vi "single sweep - next chunk - V0.vi"(4 "algorithm":string="statemachine", 5 "cursor bracket: Scan, win":refnum<vi>, 6 "mode":enum16{"first time", "uniform", "adaptive"}(ring)=enum."adaptive", 7 "Plot:response":refnum<vi>, 9 "x + iy":cdb[](array[numeric])=[0.0014961444378751654-0.005494848789731022i, 0.0014279223595474386-0.005470747752736027i, 0.001513711413730512-0.00552874878044623i, 0.001502407562898675-0.005445638194888334i, 0.0015845696982058808-0.005437153149732619i, 0.0015101628497750257-0.005522728337901211i, 0.0015131031857027845-0.005520920485579818i, 0.0015751707865244427-0.005432155579139866i, 0.001381283887581937-0.0055376532176146485i, 0.0013869914972504977-0.005471269712968517i], 10 "chunks":T1={"start F"=1400000.0, "stop F"=3000000.0, "total number of points"=6000, "chunk size"=10, "freq step (Hz)"=400.0, "update rate (Hz)"=250.0, "adaptive parameters"={"wavepacket"={"R"=0.5, "wave number"=15.0, "delta k"=7.0, "radii vector"=[], "radial section"=[], "wave vector"=22.0, "wavepacket is"=TRUE}, "number of grid points"=50, "decimation threshold"=1, "Voltage range"=0.1, "target freq step"=20.0, "target spot size"=0.05, "factor"=1.0, "another factor"=1.0, "analyze last # sec"=1, "scale factor"=10}, "total sweep time (sec)"=24.0, "chunk time (sec)"=0.04, "spot size (V)"=5.8152639158694506e-05, "uniform freq step (Hz)"=266.6666666666667, "next start freq"=1412960.0000000002} {"next start freq" format="%#_4f"; "uniform freq step (Hz)" format="%#_3f"; "spot size (V)" format="%#_2f"; "adaptive parameters"."wavepacket"."delta k" format="%#_3f"; "adaptive parameters"."wavepacket"."wave number" format="%#_3f"; "adaptive parameters"."wavepacket"."R" format="%#_3f"; "freq step (Hz)" format="%#_2f"; "stop F" format="%#_3f"; "start F" format="%#_3f"}, 11 "F Array in":dbl[](array[numeric])=[1408640.0000000002, 1408672.0000000002, 1408704.0000000002, 1408736.0000000002, 1408768.0000000002, 1408800.0000000002, 1408832.0000000002, 1408864.0000000002, 1408896.0000000002, 1408928.0000000002]) -> (0 "window":cluster{dbl[], dbl[]}[](array[cluster])=[{array[500 elements], array[500 elements]}, {array[500 elements], array[500 elements]}, {[2988000.0, 2988320.0, 2988640.0, 2992640.0, 2996640.0, 3000640.0, 3004640.0, 3004960.0, 3008960.0, 3012960.0, 3013280.0, 3013600.0, 3017600.0, 3021600.0, 3025600.0, 3029600.0, 3033600.0, 3037600.0, 3041600.0, 3045600.0, 3049600.0, 3053600.0, 3057600.0, 3061600.0, 3065600.0, 3069600.0, 3073600.0, 3077600.0, 3077920.0, 3081920.0, 3085920.0, 3089920.0, 3093920.0, 3094240.0, 3098240.0, 3102240.0, 3102560.0, 3106560.0, 3110560.0, 3114560.0, 3118560.0, 3122560.0, 3126560.0, 3126880.0, 3130880.0, 1408320.0000000002, 1408640.0000000002, 1408960.0000000002, 1412960.0000000002, 1416960.0000000002], [0.00011132389559019453, 0.00010071650784182846, 0.00011473215051580125, 0.00014782978553753255, 0.00012363182181742826, 8.247818640394286e-05, 4.853569183607435e-05, 0.00011091209952173231, 5.335161099533373e-05, 8.997863187674346e-05, 6.096859045620223e-05, 0.00011032129342938127, 0.00014137261844608594, 0.00011027777124700277, 7.83124094059187e-05, 8.359930932665522e-05, 8.923138939621333e-05, 5.1551353463386254e-05, 8.295869472945261e-05, 8.128556971740557e-05, 7.69462000730066e-05, 7.144851315975473e-05, 7.952519321081926e-05, 9.517779850815267e-05, 9.704248606160299e-05, 0.00011632633414436816, 0.00010390576558171027, 0.00010696411213824573, 9.728970607203878e-05, 0.0001308279684608251, 6.464132471543712e-05, 0.00011952708368690759, 6.148514772660781e-05, 8.068062707804084e-05, 0.00011312139911462234, 6.908047023895298e-05, 5.936822230667681e-05, 0.00010020626764101784, 0.00012946703718681504, 0.00010013466000813908, 6.912354981532708e-05, 0.00011430443059521424, 0.00012513022719631484, 0.00010923915541343698, 0.00011547570124367561, 0.003905008531492904, 0.0033917347983675613, 0.003353407371274829, 0.003173893478063239, 0.003074549188462509]}, {[2988000.0, 2988320.0, 2988640.0, 2992640.0, 2996640.0, 3000640.0, 3004640.0, 3004960.0, 3008960.0, 3012960.0, 3013280.0, 3013600.0, 3017600.0, 3021600.0, 3025600.0, 3029600.0, 3033600.0, 3037600.0, 3041600.0, 3045600.0, 3049600.0, 3053600.0, 3057600.0, 3061600.0, 3065600.0, 3069600.0, 3073600.0, 3077600.0, 3077920.0, 3081920.0, 3085920.0, 3089920.0, 3093920.0, 3094240.0, 3098240.0, 3102240.0, 3102560.0, 3106560.0, 3110560.0, 3114560.0, 3118560.0, 3122560.0, 3126560.0, 3126880.0, 3130880.0, 1408320.0000000002, 1408640.0000000002, 1408960.0000000002, 1412960.0000000002, 1416960.0000000002], [0.013694694005932529, 0.014489837272950239, 0.009503558469975002, 0.009528211653947193, 0.012476459558180022, 0.013578618032833986, 0.020768560303619083, 0.020949019291147796, 0.02034486055557658, 0.011646926818591538, 0.009458678658119484, 0.006310537358577627, 0.00038583342676350336, 0.006103250811137311, 0.001250242454873757, 0.005243640192020321, 0.008719705117003948, 0.006143859432854482, 0.006470257084291946, 0.006348276391260311, 0.008375758813583493, 0.0038044691071716097, 0.0015818509944146705, 0.003581191521982118, 0.0006892804064302445, 0.0025054554152808646, 0.004117073317010084, 0.002045540413627015, 0.0007410657254269008, 0.005324792655608368, 0.012491486267365477, 0.013829845176253889, 0.009382411909246033, 0.008531253899751555, 0.006057094794442862, 0.000802518050976467, 0.006846069080773061, 0.004537353265510852, 0.008159903085244793, 0.0028444703551188284, 0.007454427723095375, 4.4410190171195404e-05, 0.0015101954709487865, 0.004475681662266171, 0.010341490132182555, 0.01226244459723875, 0.015308020505903021, 0.005597683037877003, 0.0037965342629815418, 0.0016913227005998597]}], 1 "fancy circles":cluster{dbl[], dbl[]}[](array[cluster])=[{[0.004347976639836461, 0.0043237329011621035, 0.004251384023380436, 0.004132070991513198, 0.003967675443347089, 0.0037607899948818246, 0.0035146773532270816, 0.00323321886176232, 0.0029208532890330928, 0.002582506826719488, 0.00222351540065057, 0.0018495405200665291, 0.0014664799922359413, 0.001080374910511962, 0.0006973143826813736, 0.0003233395020973332, -3.56519239715844e-05, -0.0003739983862851902, -0.0006863639590144167, -0.0009678224504791784, -0.0012139350921339205, -0.0014208205405991845, -0.001585216088765295, -0.0017045291206325324, -0.0017768779984142003, -0.001801121737088557, -0.0017768779984142003, -0.0017045291206325324, -0.0015852160887652941, -0.001420820540599184, -0.00121393509213392, -0.000967822450479178, -0.0006863639590144162, -0.00037399838628518847, -3.5651923971582664e-05, 0.0003233395020973332, 0.0006973143826813741, 0.0010803749105119625, 0.0014664799922359426, 0.001849540520066531, 0.0022235154006505697, 0.002582506826719488, 0.0029208532890330936, 0.003233218861762321, 0.003514677353227083, 0.0037607899948818254, 0.003967675443347089, 0.004132070991513199, 0.004251384023380437, 0.0043237329011621035], [-0.00253283204245687, -0.0021474888509143563, -0.001768222751695333, -0.0014010149977470693, -0.0010516566747086093, -0.0007256573720308159, -0.00042815829345946126, -0.00016385117718095135, 6.309569569158376e-05, 0.0002491032374014545, 0.0003912379979003752, 0.0004872584271080889, 0.0005356502254961651, 0.0005356502254961651, 0.00048725842710808844, 0.0003912379979003752, 0.00024910323740145405, 6.309569569158376e-05, -0.00016385117718095135, -0.0004281582934594617, -0.0007256573720308154, -0.0010516566747086097, -0.00140101499774707, -0.0017682227516953328, -0.0021474888509143567, -0.002532832042456871, -0.002918175233999384, -0.003297441333218408, -0.003664649087166672, -0.004014007410205131, -0.004340006712882925, -0.004637505791454279, -0.004901812907732789, -0.005128759780605325, -0.005314767322315195, -0.005456902082814115, -0.0055529225120218295, -0.005601314310409906, -0.005601314310409906, -0.005552922512021829, -0.005456902082814115, -0.005314767322315195, -0.0051287597806053235, -0.004901812907732788, -0.004637505791454277, -0.004340006712882922, -0.004014007410205131, -0.0036646490871666704, -0.0032974413332184063, -0.0029181752339993822]}, {[-0.0007985969840225416, -0.0005913945404828922, -0.0003841920969432428, -0.0001769896534035934, 3.0212790136055923e-05, 0.00023741523367570524, 0.0004446176772153548, 0.0006518201207550041, 0.0008590225642946534, 0.0010662250078343027, 0.001273427451373952, 0.0014806298949136016, 0.001687832338453251, 0.0018950347819929002, 0.00210223722553255, 0.0023094396690721986, 0.002516642112611848, 0.0027238445561514977, 0.0029310469996911472, 0.003138249443230796], [-0.004804300169328853, -0.004577153356641655, -0.004350006543954456, -0.004122859731267258, -0.00389571291858006, -0.0036685661058928616, -0.003441419293205663, -0.003214272480518465, -0.0029871256678312666, -0.002759978855144068, -0.00253283204245687, -0.0023056852297696716, -0.002078538417082473, -0.0018513916043952751, -0.0016242447917080766, -0.0013970979790208786, -0.0011699511663336801, -0.0009428043536464817, -0.0007156575409592832, -0.0004885107282720852]}, {[-0.0009980406754980312, -0.0007708938628108329, -0.0005437470501236345, -0.0003166002374364362, -8.945342474923792e-05, 0.00013769338793796033, 0.0003648402006251588, 0.0005919870133123571, 0.0008191338259995553, 0.0010462806386867538, 0.0012734274513739518, 0.0015005742640611503, 0.0017277210767483488, 0.001954867889435547, 0.0021820147021227453, 0.0024091615148099433, 0.002636308327497142, 0.0028634551401843403, 0.0030906019528715387, 0.0033177487655587368], [-0.0004608076070603765, -0.0006680100506000258, -0.0008752124941396752, -0.0010824149376793247, -0.001289617381218974, -0.0014968198247586233, -0.0017040222682982728, -0.0019112247118379222, -0.0021184271553775715, -0.0023256295989172206, -0.00253283204245687, -0.0027400344859965196, -0.002947236929536169, -0.0031544393730758183, -0.003361641816615468, -0.003568844260155117, -0.0037760467036947664, -0.003983249147234416, -0.004190451590774065, -0.004397654034313714]}], 2 "chunks out":T1={"start F"=1400000.0, "stop F"=3000000.0, "total number of points"=6000, "chunk size"=10, "freq step (Hz)"=400.0, "update rate (Hz)"=250.0, "adaptive parameters"={"wavepacket"={"R"=0.5, "wave number"=15.0, "delta k"=7.0, "radii vector"=[], "radial section"=[], "wave vector"=22.0, "wavepacket is"=TRUE}, "number of grid points"=50, "decimation threshold"=1, "Voltage range"=0.1, "target freq step"=20.0, "target spot size"=0.05, "factor"=1.0, "another factor"=1.0, "analyze last # sec"=1, "scale factor"=10}, "total sweep time (sec)"=24.0, "chunk time (sec)"=0.04, "spot size (V)"=5.8152639158694506e-05, "uniform freq step (Hz)"=266.6666666666667, "next start freq"=1412960.0000000002} {"next start freq" format="%#_4f"; "uniform freq step (Hz)" format="%#_3f"; "spot size (V)" format="%#_2f"; "adaptive parameters"."wavepacket"."delta k" format="%#_3f"; "adaptive parameters"."wavepacket"."wave number" format="%#_3f"; "adaptive parameters"."wavepacket"."R" format="%#_3f"; "freq step (Hz)" format="%#_2f"; "stop F" format="%#_3f"; "start F" format="%#_3f"}, 3 "F Array":dbl[](array[numeric])=[1412960.0000000002, 1413360.0000000002, 1413760.0000000002, 1414160.0000000002, 1414560.0000000002, 1414960.0000000002, 1415360.0000000002, 1415760.0000000002, 1416160.0000000002, 1416560.0000000002])   [LabVIEW 2010]
uses:
  single sweep - frequency chunks.ctl
  single sweep - adaptive parameters.ctl
  wavepacket.ctl
  generate wave packet V2.vi
  smart decimate .vi
  set up complex region.vi
  inteference -- find center V2.vi
  find circle corners V3.vi
  linear interpolation - re.vi
  peak - phase around center.vi
  peak - simple guess at omega.vi
  peak - fix phase.vi
  peak - fit phase around center.vi
  peak - calculate lorentzian.vi
  draw a line.vi
  draw a circle.vi
  generate linear region.vi
  find circle corners - rescale back.vi
  <vilib>/Analysis/baseanly.llb/Median.vi
  <vilib>/Analysis/baseanly.llb/Mean.vi
  <vilib>/Analysis/2dsp.llb/Unwrap Phase.vi
  <vilib>/gmath/NumericalOptimization/Nonlinear Curve Fit.vi
  <vilib>/gmath/NumericalOptimization/Nonlinear Curve Fit LM.vi
  <vilib>/Utility/error.llb/Clear Errors.vi
panel:
  in  "in peak win (kHz)":dbl=0.5
  in  "in peak threshold":i32=10
  in  "search win (kHz)":dbl=12.0
  in  "scale factor":i32=3
  out "in peak threshold  ?":bool
  in  "analyze last # of secs":dbl=0.3
  out "omega(0) (kHz)":dbl=3120.5599996327037 format="%#_4f"
  in  "min speed (kHz/sec)":dbl=8.0
  in  "max speed (kHz/sec)":dbl=100.0
  out "thershold ?":bool=TRUE
  in  "threshold":dbl=20.0
  out "heater":dbl=5.77997331934377
  out "ln(x) 0":dbl=-6.907755278982137
  out "ln(x)":dbl=-9.498835202893684
  in  "negative":i32=2
  in  "I (sec)":dbl=2.0
  in  "dz0":dbl=0.001 format="%#_6f"
  in  "max dF":dbl=2000.0
  in  "min dF":dbl=20.0
  in  "P":dbl=2.0
  out "32bit integer":i32=50
  out "above ?":bool
  in  "V":dbl=0.05
  in  "factor":dbl=0.8
  out "r":dbl
  out "viscosity":dbl
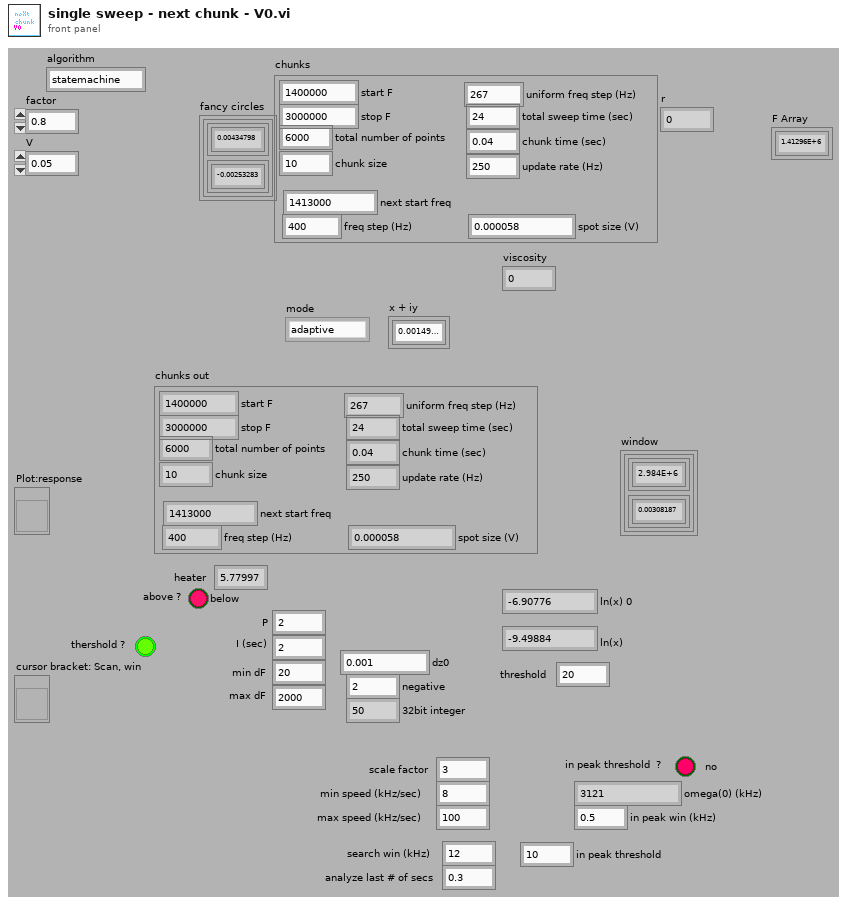
[diagram p1: front panel]
types:
  T1 = typedef "single sweep - frequency chunks.ctl" = cluster{"start F":dbl, "stop F":dbl, "total number of points":i32, "chunk size":i32, "freq step (Hz)":dbl, "update rate (Hz)":dbl, "adaptive parameters":T2, "total sweep time (sec)":dbl, "chunk time (sec)":dbl, "spot size (V)":dbl, "uniform freq step (Hz)":dbl, "next start freq":dbl}
  T2 = typedef "single sweep - adaptive parameters.ctl" = cluster{"wavepacket":T3, "number of grid points":i32, "decimation threshold":i32, "Voltage range":dbl, "target freq step":dbl, "target spot size":dbl, "factor":dbl, "another factor":dbl, "analyze last # sec":i32, "scale factor":i32}
  T3 = typedef "wavepacket.ctl" = cluster{"R":dbl, "wave number":dbl, "delta k":dbl, "radii vector":dbl[], "radial section":cdb[], "wave vector":dbl, "wavepacket is":bool}
  T4 = enum16{"", "cursor moves", "center change", "window change", "init", "check", "reset", "set y to middle"}
  T5 = typedef "circle corners.ctl" = cluster{"z (-pi/2)":cdb, "z(inf)":cdb, "z (pi/2)":cdb, "z center":cdb, "z(0)":cdb, "radius":dbl}
  T6 = typedef "lorentzian.ctl" = cluster{"Amplitude":dbl, "omega(0)":dbl, "Gamma":dbl, "phase":dbl, "Q":dbl, "Norm  Ampl":dbl, "z (inf)":cdb, "4corners":T5}
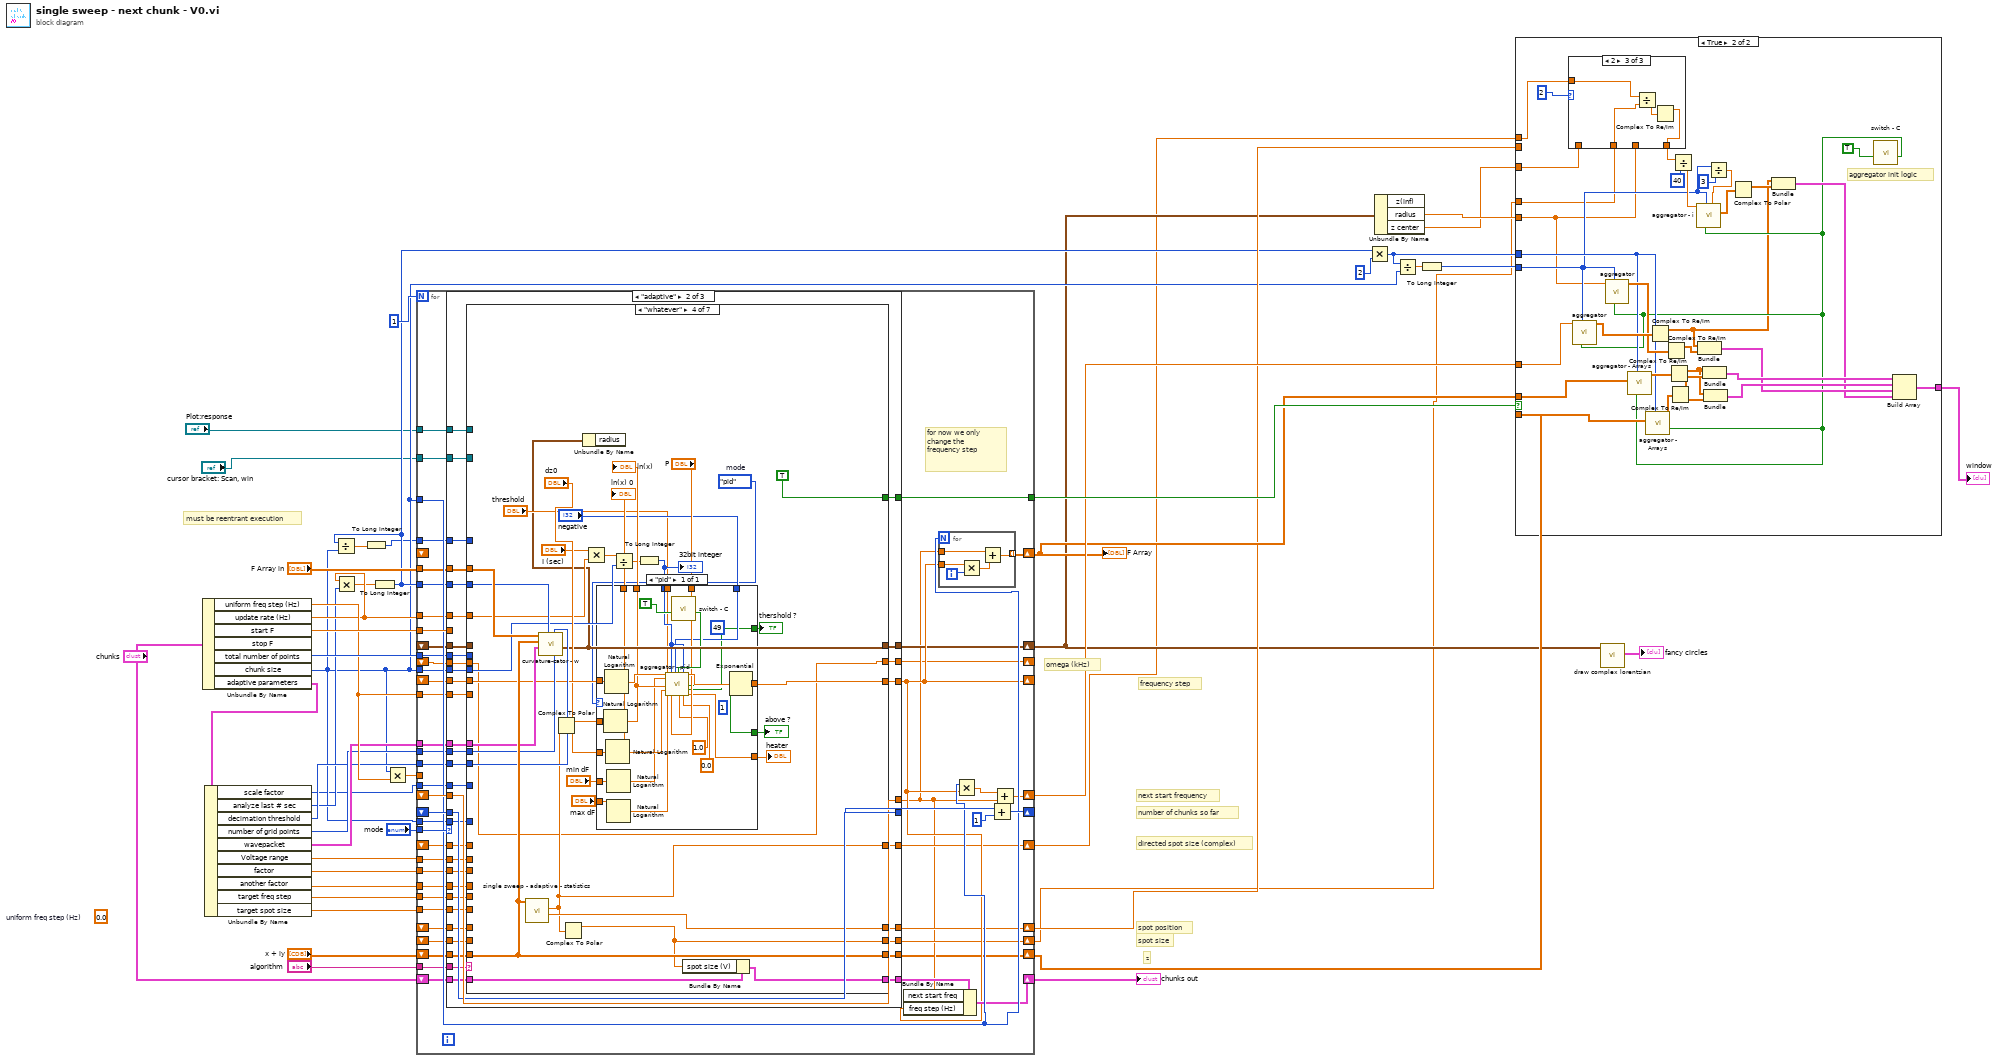
[diagram p0: block diagram]
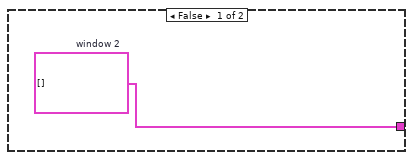
[diagram p2: hidden frame]
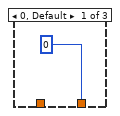
[diagram p3: hidden frame]
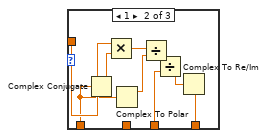
[diagram p4: hidden frame]
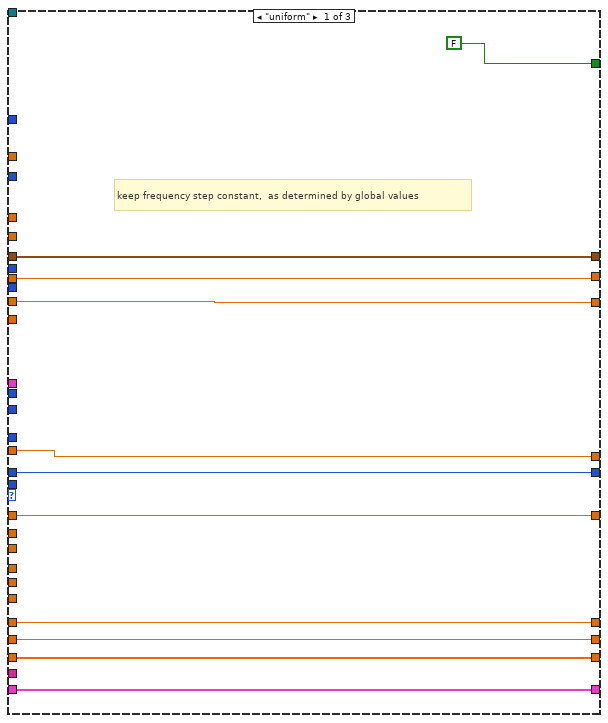
[diagram p5: hidden frame]
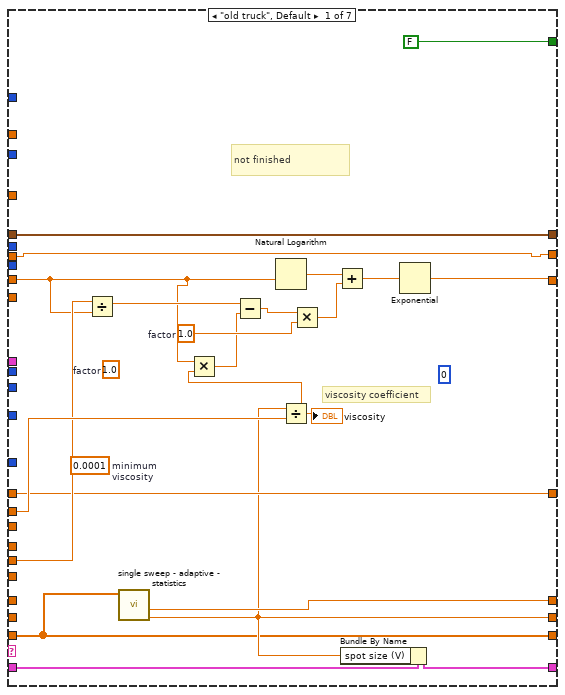
[diagram p6: hidden frame]
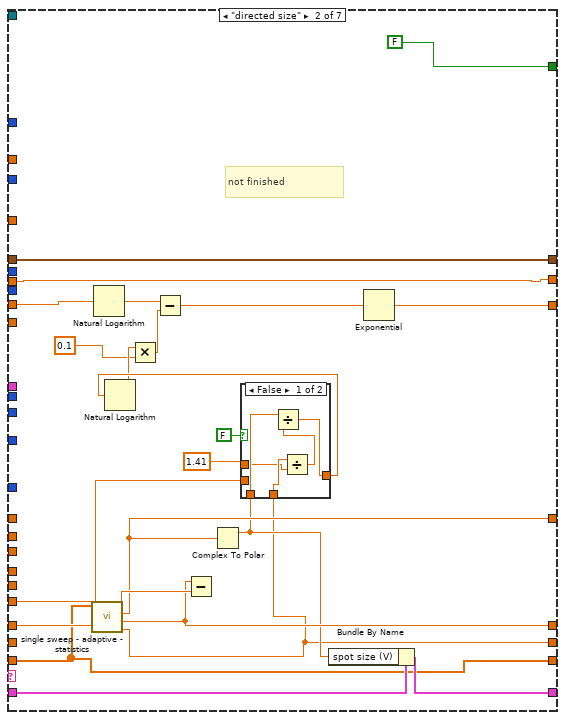
[diagram p7: hidden frame]
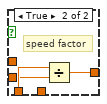
[diagram p8: hidden frame]
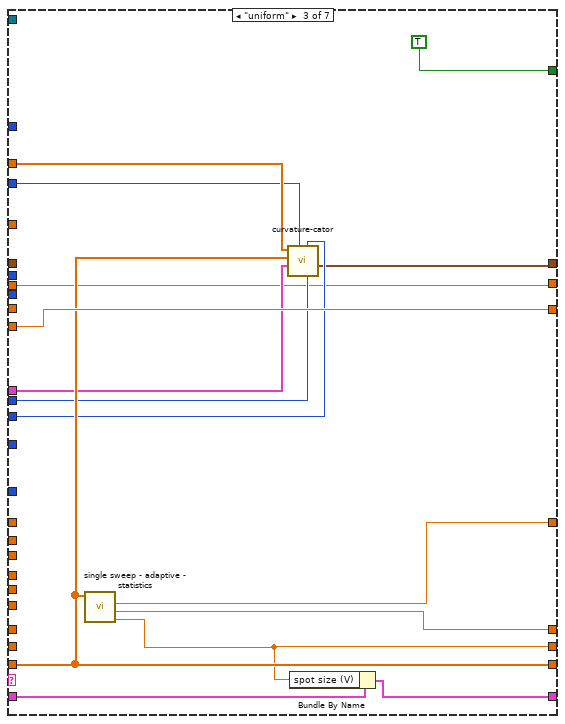
[diagram p9: hidden frame]
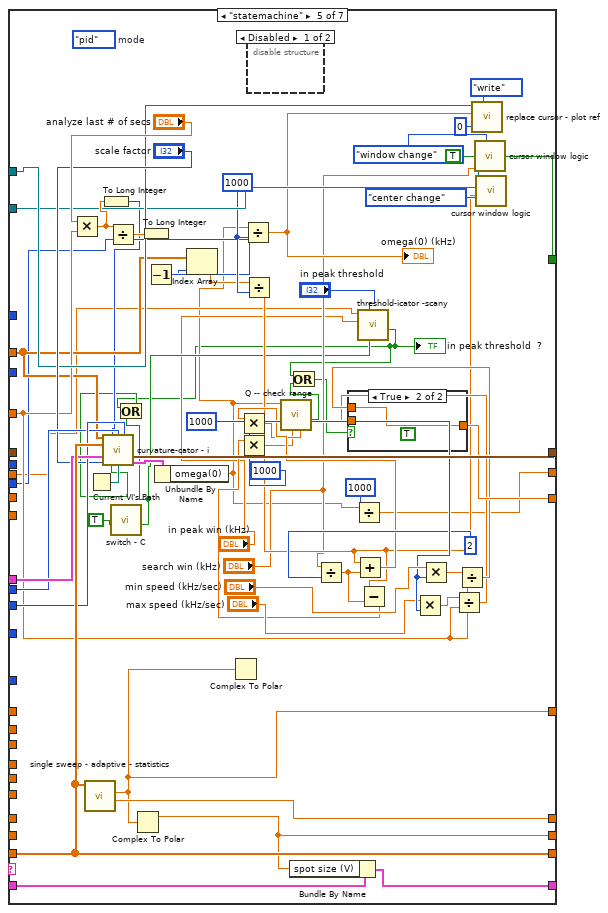
[diagram p10: hidden frame]
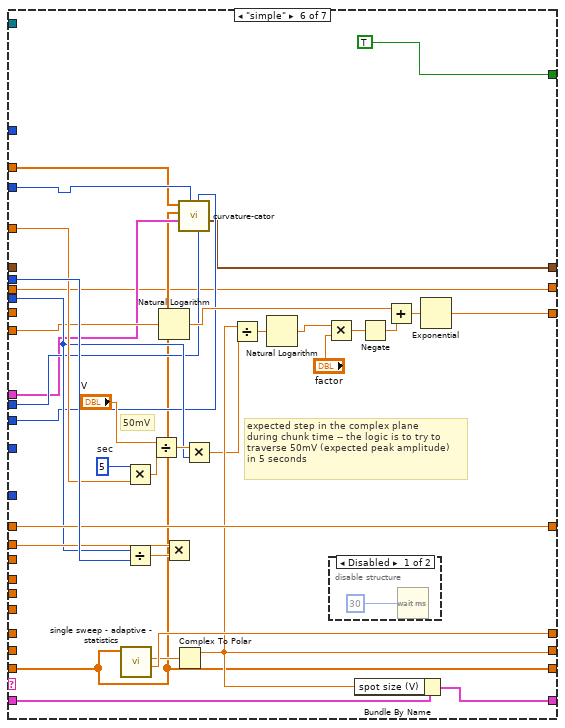
[diagram p13: hidden frame]
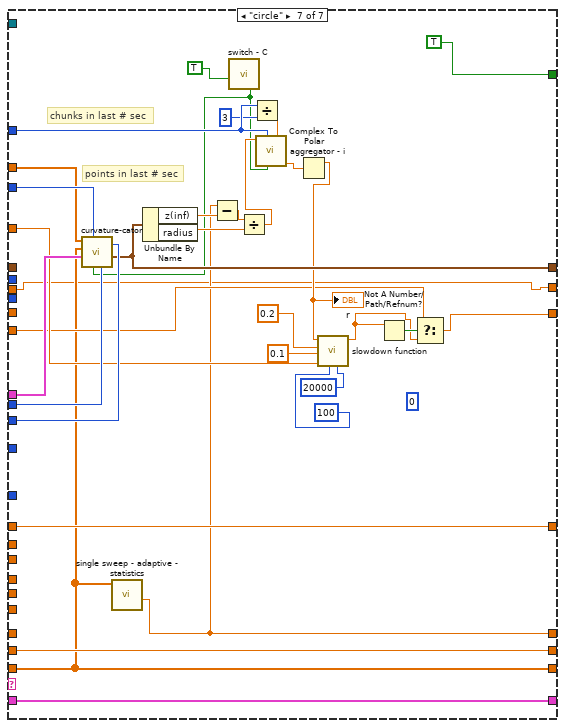
[diagram p15: hidden frame]
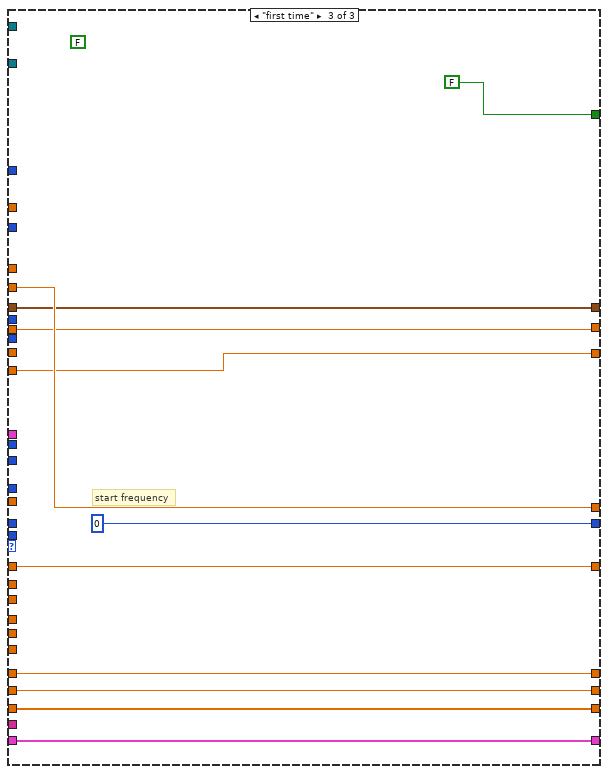
[diagram p16: hidden frame]
diagram:
  (unwired) 0.0  # uniform freq step (Hz)
  # "omega (kHz)"
  # "z"
  # "must be reentrant execution"
  # "directed spot size (complex)"
  # "spot position"
  # "spot size"
  # "frequency step"
  # "number of chunks so far"
  # "next start frequency"
  n1 = Unbundle By Name("chunks") -> ("uniform freq step (Hz)"=w31:dbl, "update rate (Hz)"=w29:dbl, "start F"=w44:dbl, "total number of points"=w40:i32, "chunk size"=w11:i32, "adaptive parameters"=w37:T2)  [unwired: 1 out]
  n2 = Unbundle By Name(w37) -> ("scale factor"=w3:i32, "analyze last # sec"=w25:i32, "decimation threshold"=w26:i32, "number of grid points"=w27:i32, "wavepacket"=w28:T3, "Voltage range"=w33:dbl, "factor"=w35:dbl, "another factor"=w34:dbl, "target freq step"=w36:dbl, "target spot size"=w32:dbl)
  n3 = Multiply(x=w29, y=w25) -> (x*y=w23:dbl)
  n4 = To Long Integer(number=w23) -> (32bit integer=w12:i32)
  n5 = Divide(x=w12, y=w11) -> (x/y=w10:dbl)
  n6 = To Long Integer(number=w10) -> (32bit integer=w9:i32)
  n7 = Multiply(x=w11, y=w31) -> (x*y=w45:dbl)
  n8 = for {
    N: 1 -> [_]
    tunnel: w31 -> [w66]
    tunnel: w11 -> [w88]
    tunnel: "mode" -> [w96]
    shift-right: [w56] -> w22
    shift-left: _ -> [w94]
    shift-right: [w91] -> _
    shift-left: _ -> [w93]
    tunnel: w45 -> [_]
    tunnel: w44 -> [w89]
    shift-right: [w95] -> w20
    shift-left: _ -> [_]
    tunnel: "F Array in" -> [w85]
    tunnel: w11 -> [w84]
    tunnel: w40 -> [w83]
    tunnel: w33 -> [w82]
    shift-right: [w81] -> w39
    shift-left: "chunks" -> [w76]
    shift-right: [w80] -> _
    shift-left: _ -> [w79]
    tunnel: "algorithm" -> [w78]
    tunnel: w36 -> [w77]
    shift-right: [w74] -> w4
    shift-left: _ -> [w71]
    shift-right: [w73] -> w13
    shift-left: _ -> [w72]
    tunnel: w11 -> [w70]
    shift-right: [w69] -> w6
    shift-left: _ -> [w67]
    tunnel: w32 -> [w68]
    tunnel: w35 -> [w65]
    tunnel: w34 -> [w64]
    tunnel: w29 -> [w63]
    tunnel: w12 -> [w62]
    tunnel: w28 -> [w61]
    tunnel: w27 -> [w60]
    tunnel: w26 -> [w59]
    shift-right: [w58] -> w7
    shift-left: _ -> [w57]
    tunnel: [w53] -> w24
    shift-right: [w54] -> w18
    shift-left: "x + iy" -> [w86]
    tunnel: w9 -> [w52]
    tunnel: w3 -> [w51]
    tunnel: "cursor bracket: Scan, win" -> [w50]
    tunnel: "Plot:response" -> [w49]
    shift-right: [w48] -> _
    shift-left: _ -> [w47]
    # "for now we only change the \nfrequency step"
    n9 = case shown="\"adaptive\"" w96 {
      tunnel: [w107 w146 w411] -> w55
      tunnel: [w105 w145 0] -> w92
      tunnel: w94 -> [w107 w146 _]
      tunnel: w93 -> [w105 w145 _]
      tunnel: w89 -> [_ _ w411]
      tunnel: [w106 w143 w406] -> w80
      tunnel: w79 -> [w106 w144 _]
      tunnel: w86 -> [w98 w142 w403]
      tunnel: w85 -> [_ w141 _]
      tunnel: w84 -> [_ w140 _]
      tunnel: w83 -> [_ w139 _]
      tunnel: w82 -> [_ w138 _]
      tunnel: w78 -> [_ w137 _]
      tunnel: w77 -> [_ w136 _]
      tunnel: w76 -> [w104 w135 w410]
      tunnel: [w104 w134 w410] -> w75
      tunnel: [w102 w133 w408] -> w74
      tunnel: [w103 w132 w409] -> w73
      tunnel: w72 -> [w103 w131 w409]
      tunnel: w71 -> [w102 w130 w408]
      tunnel: w70 -> [_ w129 _]
      tunnel: [w101 w128 w407] -> w69
      tunnel: w68 -> [_ w127 _]
      tunnel: w67 -> [w101 w126 w407]
      tunnel: w66 -> [_ w123 w406]
      tunnel: w65 -> [_ w125 _]
      tunnel: w64 -> [_ w124 _]
      tunnel: w63 -> [_ w122 _]
      tunnel: w62 -> [_ w121 _]
      tunnel: w61 -> [_ w120 _]
      tunnel: w60 -> [_ w119 _]
      tunnel: w59 -> [_ w118 _]
      tunnel: [w100 w117 w405] -> w58
      tunnel: w57 -> [w100 w116 w405]
      tunnel: [FALSE w115 FALSE] -> w53
      tunnel: [w98 w114 w403] -> w54
      tunnel: w52 -> [_ w113 _]
      tunnel: w51 -> [_ w112 _]
      tunnel: w50 -> [_ w111 _]
      tunnel: w49 -> [_ w110 _]
      tunnel: [w97 w109 w402] -> w48
      tunnel: w47 -> [w97 w108 w402]
      frame "uniform" {
        # "keep frequency step constant,  as determined by global values"
      }
      frame "adaptive" {
        n10 = case shown="\"whatever\"" w137 {
          tunnel: w144 -> [w154 w180 _ w238 _ _ _]
          tunnel: [w157 w179 w212 w237 w317 w351 w373] -> w143
          tunnel: w142 -> [w148 w169 w208 w245 w330 w336 w372]
          tunnel: w141 -> [_ _ w209 w246 w288 w340 w397]
          tunnel: w140 -> [_ _ _ w225 w286 w353 _]
          tunnel: w139 -> [_ _ _ _ _ w366 _]
          tunnel: w138 -> [w163 _ _ _ _ w365 _]
          tunnel: w136 -> [w162 _ _ _ _ _ _]
          tunnel: w135 -> [w165 w189 w199 w239 w324 w363 w401]
          tunnel: [w164 w188 w200 w240 w325 w364 w401] -> w134
          tunnel: [w151 w174 w201 w231 w322 w359 w400] -> w133
          tunnel: [w152 w186 w211 w247 w331 w361 w371] -> w132
          tunnel: w131 -> [_ w187 _ _ _ _ _]
          tunnel: w130 -> [_ _ _ _ _ _ w400]
          tunnel: w129 -> [_ _ _ _ _ _ _]
          tunnel: [w153 w185 w210 w232 w323 w362 w399] -> w128
          tunnel: w127 -> [_ w183 _ _ _ _ _]
          tunnel: w126 -> [w153 _ _ _ _ w362 w399]
          tunnel: w125 -> [_ _ _ _ _ _ _]
          tunnel: w124 -> [_ _ _ _ _ _ _]
          tunnel: w123 -> [_ _ w212 _ _ w344 w374]
          tunnel: w122 -> [_ _ _ w222 w298 w357 w382]
          tunnel: w121 -> [_ _ w204 w226 _ w341 w398]
          tunnel: w120 -> [_ _ w207 w244 w329 w339 w396]
          tunnel: w119 -> [_ _ w205 w242 w327 w342 w395]
          tunnel: w118 -> [_ _ w206 w243 w328 w343 w394]
          tunnel: [w150 w171 w202 w216 w320 w338 w388] -> w117
          tunnel: w116 -> [w150 w171 _ _ _ _ _]
          tunnel: [FALSE FALSE TRUE TRUE TRUE TRUE TRUE] -> w115
          tunnel: [w148 w169 w208 w245 w330 w336 w372] -> w114
          tunnel: w113 -> [_ _ _ _ _ _ w391]
          tunnel: w112 -> [_ _ _ _ _ _ _]
          tunnel: w111 -> [_ _ _ _ w310 _ _]
          tunnel: w110 -> [_ _ _ _ w313 _ _]
          tunnel: [w147 w168 w198 w213 w274 w334 w369] -> w109
          tunnel: w108 -> [w147 w168 w198 w213 w279 w334 w369]
          frame "old truck", Default {
            (unwired) 0
            (unwired) 1.0  # factor
            w160 = 1.0  # factor
            (unwired) 0.0001  # minimum  viscosity
            # "not finished"
            # "viscosity coefficient"
            n11 = Divide(x=w162, y=w154) -> (x/y=w161:dbl)
            n12 = call "single sweep - adaptive - statistics.vi"("x + iy"=w148) -> ("spot size"=w151:dbl, "spot position"=w152:cdb)  [unwired: 8 in, 1 out]
            n13 = Natural Logarithm(1:w154) -> (0:w159:dbl)
            n14 = Divide(x=w151, y=w163) -> (x/y=w156:dbl)
            "viscosity" <- w156
            n15 = Multiply(x=w154, y=w156) -> (x*y=w155:dbl)
            n16 = Subtract(x=w161, y=w155) -> (x-y=w167:dbl)
            n17 = Multiply(x=w167, y=w160) -> (x*y=w166:dbl)
            n18 = Add(x=w159, y=w166) -> (x+y=w158:dbl)
            n19 = Bundle By Name(cluster=w165, "spot size (V)"=w151) -> (w164:T1)
            n20 = Exponential(1:w158) -> (0:w157:dbl)
          }
          frame "directed size" {
            # "not finished"
            n21 = call "single sweep - adaptive - statistics.vi"("x + iy"=w169) -> ("spot size"=w174:dbl, "spot position"=w186:cdb, "spot directed size"=w185:cdb)  [unwired: 8 in]
            n22 = Natural Logarithm(1:w180) -> (0:w182:dbl)
            n23 = Subtract(x=w186, y=w187) -> ()  [unwired: 1 out]
            n24 = Complex To Polar(r * e^(i*theta)=w185) -> (r=w184:dbl)  [unwired: 1 out]
            n25 = case shown="False" FALSE {
              tunnel: w184 -> [w194 w197]
              tunnel: w183 -> [_ w196]
              tunnel: [w193 w195] -> w178
              tunnel: w174 -> [w192 _]
              tunnel: 1.41 -> [w190 _]
              frame False {
                n26 = Divide(x=w192, y=w190) -> (x/y=w191:dbl)
                n27 = Divide(x=w194, y=w191) -> (x/y=w193:dbl)
              }
              frame True {
                # "speed factor"
                n28 = Divide(x=w197, y=w196) -> (x/y=w195:dbl)
              }
            }
            n29 = Natural Logarithm(1:w178) -> (0:w177:dbl)
            n30 = Multiply(x=w177, y=0.1) -> (x*y=w176:dbl)
            n31 = Subtract(x=w182, y=w176) -> (x-y=w181:dbl)
            n32 = Bundle By Name(cluster=w189, "spot size (V)"=w184) -> (w188:T1)
            n33 = Exponential(1:w181) -> (0:w179:dbl)
          }
          frame "uniform" {
            n34 = call "single sweep - adaptive - statistics.vi"("x + iy"=w208) -> ("spot size"=w201:dbl, "spot position"=w211:cdb, "spot directed size"=w210:cdb)  [unwired: 8 in]
            n35 = call "curvature-cator.vi"("number of grid points"=w205, "decimation threshold"=w206, "size"=w204, "wavepacket in"=w207, "z array in"=w208, "omega array in"=w209) -> ("4 corners out"=w202:T5)  [unwired: 3 in, 2 out]
            n36 = Bundle By Name(cluster=w199, "spot size (V)"=w201) -> (w200:T1)
          }
          frame "whatever" {
            w214 = enum16{"pid"}."pid"  # mode
            n37 = call "single sweep - adaptive - statistics.vi"("x + iy"=w245) -> ("spot position"=w247:cdb, "spot directed size"=w232:cdb)  [unwired: 8 in, 1 out]
            n38 = call "curvature-cator - w.vi"("number of grid points"=w242, "decimation threshold"=w243, "size"=w226, "wavepacket in"=w244, "z array in"=w245, "omega array in"=w246) -> ("4 corners out"=w216:T5)  [unwired: 3 in, 2 out]
            n39 = Complex To Polar(r * e^(i*theta)=w232) -> (r=w215:dbl)  [unwired: 1 out]
            n40 = Complex To Polar(r * e^(i*theta)=w232) -> (r=w231:dbl)  [unwired: 1 out]
            n41 = Unbundle By Name(w216) -> ()  [unwired: 1 out]
            n42 = Multiply(x="I (sec)", y=w222) -> (x*y=w221:dbl)
            n43 = Divide(x=w221, y=w225) -> (x/y=w227:dbl)
            n44 = To Long Integer(number=w227) -> (32bit integer=w224:i32)
            "32bit integer" <- w224
            n45 = case shown="\"pid\"" w214 {
              tunnel: w238 -> [w270]
              tunnel: [w267] -> w237
              tunnel: [w264] -> w236
              tunnel: "dz0" -> [w263]
              tunnel: [w262] -> w234
              tunnel: "P" -> [w261]
              tunnel: "min dF" -> [w259]
              tunnel: "max dF" -> [w258]
              tunnel: [w255] -> w228
              tunnel: w224 -> [w254]
              tunnel: "negative" -> [w252]
              tunnel: [w251] -> w219
              tunnel: "threshold" -> [w250]
              tunnel: [w249] -> w217
              tunnel: w215 -> [w248]
              frame "pid" {
                (unwired) 1 ("y")
                (unwired) 49 ("y")
                n46 = Natural Logarithm(1:w248) -> (0:w264:dbl)
                n47 = Natural Logarithm(1:w270) -> (0:w269:dbl)
                n48 = Natural Logarithm(1:w263) -> (0:w262:dbl)
                n49 = Natural Logarithm(1:w259) -> (0:w257:dbl)
                n50 = Natural Logarithm(1:w258) -> (0:w256:dbl)
                n51 = call "switch - C.vi"("switch"=TRUE) -> ("result"=w265:bool)  [unwired: 10 in]
                n52 = call "aggregator - pid.vi"("df"=w269, "low"=w257, "threshold"=w250, "dz"=w264, "dz0"=w262, "high"=w256, "requested size"=w254, "P"=w261, "negative"=w252, "first time"=w265, "I"=1.0 ("y"), "requested averaging interval"=w254, "D"=0.0 ("y")) -> ("new df"=w268:dbl, "above ?"=w255:bool, "thershold ?"=w249:bool, "heater"=w251:dbl)  [unwired: 3 in]
                n53 = Exponential(1:w268) -> (0:w267:dbl)
              }
            }
            "above ?" <- w228
            "ln(x)" <- w236
            "ln(x) 0" <- w234
            "heater" <- w219
            "thershold ?" <- w217
            n54 = Bundle By Name(cluster=w239, "spot size (V)"=w231) -> (w240:T1)
          }
          frame "statemachine" {
            w293 = 1000
            w300 = 1000
            w306 = 1000
            (unwired) enum16{"pid"}."pid"  # mode
            n55 = Multiply(x="analyze last # of secs", y=w298) -> (x*y=w315:dbl)
            n56 = call "single sweep - adaptive - statistics.vi"("x + iy"=w330) -> ("spot position"=w331:cdb, "spot directed size"=w323:cdb)  [unwired: 8 in, 1 out]
            n57 = Current VI's Path() -> (path=w319:path)
            n58 = To Long Integer(number=w315) -> (32bit integer=w284:i32)
            n59 = Divide(x=w315, y=w286) -> (x/y=w321:dbl)
            n60 = call "switch - C.vi"("switch"=TRUE) -> ("result"=w280:bool)  [unwired: 10 in]
            n61 = Complex To Polar(r * e^(i*theta)=w323) -> (r=w322:dbl)  [unwired: 1 out]
            n62 = To Long Integer(number=w321) -> ()  [unwired: 1 out]
            n63 = Decrement(x=w286) -> (x-1=w285:i32)
            n64 = Index Array(array=w288, index=w285) -> (element=w287:dbl)
            n65 = Complex To Polar(r * e^(i*theta)=w323) -> ()  [unwired: 2 out]
            n66 = Divide(x=w287, y=w306) -> (x/y=w289:dbl)
            n67 = disable-structure shown="Disabled" {
              frame Disabled {
              }
              frame Enabled {
              }
            }
            n68 = Bundle By Name(cluster=w324, "spot size (V)"=w322) -> (w325:T1)
            n69 = Divide(x="search win (kHz)", y=2) -> (x/y=w295:dbl)
            n70 = Add(x=w289, y=w295) -> (x+y=w294:dbl)
            n71 = Multiply(x=w294, y=w293) -> (x*y=w291:dbl)
            n72 = call "threshold-icator -scany.vi"("first time"=w280, "requested size"="in peak threshold", "gamma"="in peak win (kHz)", "omega"=w279) -> ("new peak"=w272:bool)  [unwired: 4 in, 3 out]
            "in peak threshold  ?" <- w272
            n73 = Or(x=w272, y=w280) -> (x .or. y?=w278:bool)
            n74 = call "curvature-cator - i.vi"("omega array in"=w288, "size"=w284, "number of grid points"=w327, "decimation threshold"=w328, "z array in"=w330, "wavepacket in"=w329, "scale factor"="scale factor", "first time"=w278, "main VI path"=w319) -> ("4 corners rescaled out"=w320:T5, "lorentzian out"=w318:T6)  [unwired: 3 in, 2 out]
            n75 = Unbundle By Name(w318) -> ("omega(0)"=w275:dbl)
            n76 = Divide(x=w275, y=w306) -> (x/y=w305:dbl)
            "omega(0) (kHz)" <- w305
            n77 = Divide(x=w275, y=1000) -> (x/y=w274:dbl)
            n78 = Subtract(x=w289, y=w295) -> (x-y=w292:dbl)
            n79 = Multiply(x=w292, y=w293) -> (x*y=w290:dbl)
            n80 = call "Q -- check range.vi"("upper"=w291, "lower"=w290, "number"=w275) -> ("in range?"=w273:bool)  [unwired: 4 in, 4 out]
            n81 = Or(x=w272, y=w273) -> (x .or. y?=w271:bool)
            n82 = Multiply(x="max speed (kHz/sec)", y=w300) -> (x*y=w301:dbl)
            n83 = Multiply(x="min speed (kHz/sec)", y=w300) -> (x*y=w303:dbl)
            n84 = Divide(x=w301, y=w298) -> (x/y=w297:dbl)
            n85 = Divide(x=w303, y=w298) -> (x/y=w302:dbl)
            n86 = case shown="True" w271 {
              tunnel: [w332 w333] -> w317
              tunnel: w302 -> [_ w333]
              tunnel: w297 -> [w332 _]
              frame False {
              }
              frame True {
                (unwired) TRUE
              }
            }
            n87 = call "replace cursor - plot ref.vi"("action"=enum16{"", "read", "write"}."write", "cursor index"=0, "new X"=w305, "Plot ref in"=w313) -> ()  [unwired: 5 in, 3 out]
            n88 = call "cursor window logic.vi"("action"=T4."center change", "center"=w289, "cursor bracket in"=w310) -> ("cursor bracket out"=w308:refnum<vi>)  [unwired: 7 in, 1 out]
            n89 = call "cursor window logic.vi"("action"=T4."window change", "window"="search win (kHz)", "cursor bracket in"=w308) -> ()  [unwired: 7 in, 2 out]
          }
          frame "simple" {
            w358 = 5  # sec
            # "expected step in the complex plane \nduring chunk time -- the logic is to try to \ntraverse 50mV (expected peak amplitude)\nin 5 seconds"
            # "50mV"
            n90 = call "single sweep - adaptive - statistics.vi"("x + iy"=w336) -> ("spot position"=w361:cdb, "spot directed size"=w360:cdb)  [unwired: 8 in, 1 out]
            n91 = Multiply(x=w358, y=w357) -> (x*y=w355:dbl)
            n92 = Divide(x=w353, y=w366) -> (x/y=w367:dbl)
            n93 = Divide(x="V", y=w355) -> (x/y=w354:dbl)
            n94 = Natural Logarithm(1:w344) -> (0:w345:dbl)
            n95 = Multiply(x=w365, y=w367) -> ()  [unwired: 1 out]
            n96 = Complex To Polar(r * e^(i*theta)=w360) -> (r=w359:dbl)  [unwired: 1 out]
            n97 = call "curvature-cator.vi"("number of grid points"=w342, "decimation threshold"=w343, "size"=w341, "wavepacket in"=w339, "z array in"=w336, "omega array in"=w340) -> ("4 corners out"=w338:T5)  [unwired: 3 in, 2 out]
            n98 = Multiply(x=w354, y=w353) -> (x*y=w352:dbl)
            n99 = Divide(x=w359, y=w352) -> (x/y=w335:dbl)
            n100 = Natural Logarithm(1:w335) -> (0:w350:dbl)
            n101 = Multiply(x=w350, y="factor") -> (x*y=w348:dbl)
            n102 = disable-structure shown="Disabled" {
              frame Disabled {
                n103 = Wait (ms)(milliseconds to wait=u32 30) -> ()  [unwired: 1 out]
              }
              frame Enabled {
              }
            }
            n104 = Bundle By Name(cluster=w363, "spot size (V)"=w359) -> (w364:T1)
            n105 = Negate(x=w348) -> (-x=w346:dbl)
            n106 = Add(x=w345, y=w346) -> (x+y=w347:dbl)
            n107 = Exponential(1:w347) -> (0:w351:dbl)
          }
          frame "circle" {
            (unwired) 0
            # "chunks in last # sec"
            # "points in last # sec"
            n108 = call "single sweep - adaptive - statistics.vi"("x + iy"=w372) -> ("spot position"=w371:cdb)  [unwired: 8 in, 2 out]
            n109 = call "switch - C.vi"("switch"=TRUE) -> ("result"=w370:bool)  [unwired: 10 in]
            n110 = call "curvature-cator.vi"("number of grid points"=w395, "decimation threshold"=w394, "first time"=w370, "size"=w398, "wavepacket in"=w396, "z array in"=w372, "omega array in"=w397) -> ("4 corners out"=w388:T5)  [unwired: 2 in, 2 out]
            n111 = Unbundle By Name(w388) -> ("z(inf)"=w387:cdb, "radius"=w386:dbl)
            n112 = Subtract(x=w371, y=w387) -> (x-y=w385:cdb)
            n113 = Divide(x=w385, y=w386) -> (x/y=w384:cdb)
            n114 = Divide(x=w391, y=3) -> (x/y=w390:dbl)
            n115 = call "aggregator - i.vi"("requested averaging interval"=w390, "first time"=w370, "requested size"=w391, "number"=w384) -> ("interpolated average"=w383:cdb)  [unwired: 3 in, 4 out]
            n116 = Complex To Polar(r * e^(i*theta)=w383) -> (r=w381:dbl)  [unwired: 1 out]
            "r" <- w381
            n117 = call "slowdown function.vi"("max speed"=20000, "min speed"=100, "update rate"=w382, "width"=0.1, "threshold"=0.2, "lambda"=w381) -> ("freq step"=w375:dbl)  [unwired: 5 in]
            n118 = Not A Number/Path/Refnum?(number/path/refnum=w375) -> (NaN/Path/Refnum?=w376:bool)
            n119 = Select(t=w374, s=w376, f=w375) -> (s? t:f=w373:dbl)
          }
        }
      }
      frame "first time" {
        (unwired) FALSE
        # "start frequency"
      }
    }
    n120 = Bundle By Name(cluster=w75, "next start freq"=w55, "freq step (Hz)"=w80) -> (w81:T1)
    n121 = for {
      N: w88 -> [_]
      tunnel: w80 -> [w417]
      tunnel: [w415] -> w95 mode=indexing
      tunnel: w55 -> [w413]
      i -> [w414]
      n122 = Multiply(x=w417, y=w414) -> (x*y=w416:dbl)
      n123 = Add(x=w413, y=w416) -> (x+y=w415:dbl)
    }
    n124 = Multiply(x=w88, y=w80) -> (x*y=w87:dbl)
    n125 = Add(x=w92, y=1) -> (x+y=w91:i32)
    n126 = Add(x=w87, y=w55) -> (x+y=w56:dbl)
  }
  "F Array" <- w20
  "chunks out" <- w39
  n127 = Multiply(x=w12, y=2) -> (x*y=w19:i32)
  n128 = Unbundle By Name(w7) -> ("radius"=w14:dbl, "z center"=w5:cdb)  [unwired: 1 out]
  n129 = Divide(x=w19, y=w11) -> (x/y=w15:dbl)
  n130 = To Long Integer(number=w15) -> (32bit integer=w16:i32)
  n131 = case shown="True" w24 {
    tunnel: w16 -> [_ w427]
    tunnel: w14 -> [_ w422]
    tunnel: w22 -> [_ w451]
    tunnel: w20 -> [_ w450]
    tunnel: w19 -> [_ w437]
    tunnel: w18 -> [_ w438]
    tunnel: [w418 w440] -> w17
    tunnel: w13 -> [_ _]
    tunnel: w6 -> [_ w424]
    tunnel: w5 -> [_ w423]
    tunnel: w4 -> [_ w419]
    frame False {
      w418 = cluster{dbl[], dbl[]}[] []  # window 2
    }
    frame True {
      # "aggregator init logic"
      n132 = case shown="2" 2 {
        tunnel: w424 -> [_ w461 w463]
        tunnel: w423 -> [_ w459 _]
        tunnel: w422 -> [_ w455 _]
        tunnel: [0 w453 w462] -> w421
        tunnel: w419 -> [_ _ w464]
        frame 0, Default {
        }
        frame 1 {
          n133 = Complex Conjugate(1:w459) -> (0:w460:cdb)
          n134 = Multiply(x=w461, y=w460) -> (x*y=w458:cdb)
          n135 = Complex To Polar(r * e^(i*theta)=w459) -> (r=w457:dbl)  [unwired: 1 out]
          n136 = Divide(x=w458, y=w457) -> (x/y=w456:cdb)
          n137 = Divide(x=w456, y=w455) -> (x/y=w454:cdb)
          n138 = Complex To Re/Im(x + iy=w454) -> (y=w453:dbl)  [unwired: 1 out]
        }
        frame 2 {
          n139 = Divide(x=w463, y=w464) -> (x/y=w465:cdb)
          n140 = Complex To Re/Im(x + iy=w465) -> (x=w462:dbl)  [unwired: 1 out]
        }
      }
      n141 = Divide(x=w421, y=40) -> (x/y=w434:dbl)
      n142 = Divide(x=w427, y=3) -> (x/y=w429:dbl)
      n143 = call "switch - C.vi"("switch"=TRUE) -> ("result"=w428:bool)  [unwired: 10 in]
      n144 = call "aggregator.vi"("first time"=w428, "requested size"=w427, "number"=w451) -> ("Array"=w443:cdb[])  [unwired: 8 in]
      n145 = call "aggregator.vi"("first time"=w428, "requested size"=w427, "number"=w422) -> ("Array"=w442:cdb[])  [unwired: 8 in]
      n146 = call "aggregator - Arrays.vi"("first time"=w428, "requested size"=w437, "Array in"=w450) -> ("Array"=w449:cdb[])  [unwired: 8 in]
      n147 = call "aggregator - Arrays.vi"("first time"=w428, "requested size"=w437, "Array in"=w438) -> ("Array"=w448:cdb[])  [unwired: 8 in]
      n148 = Complex To Re/Im(x + iy=w443) -> (x=w426:dbl[])  [unwired: 1 out]
      n149 = Complex To Re/Im(x + iy=w442) -> (x=w441:dbl[])  [unwired: 1 out]
      n150 = Complex To Re/Im(x + iy=w449) -> (x=w436:dbl[])  [unwired: 1 out]
      n151 = Complex To Re/Im(x + iy=w448) -> (x=w447:dbl[], y=w446:dbl[])
      n152 = call "aggregator - i.vi"("requested averaging interval"=w429, "first time"=w428, "requested size"=w427, "number"=w434) -> ("interp array"=w425:cdb[])  [unwired: 3 in, 4 out]
      n153 = Bundle(w426, w441) -> (w439:cluster{dbl[], dbl[]})  [unwired: 1 out]
      n154 = Bundle(w436, w447) -> (w445:cluster{dbl[], dbl[]})  [unwired: 1 out]
      n155 = Bundle(w436, w446) -> (w444:cluster{dbl[], dbl[]})  [unwired: 1 out]
      n156 = Complex To Polar(r * e^(i*theta)=w425) -> (r=w433:dbl[])  [unwired: 1 out]
      n157 = Bundle(w426, w433) -> (w432:cluster{dbl[], dbl[]})  [unwired: 1 out]
      n158 = Build Array(w445, w444, w439, w432) -> (w440:cluster{dbl[], dbl[]}[])
    }
  }
  "window" <- w17
  n159 = call "draw complex lorentzian.vi"("4 corners"=w7) -> ("fancy circles"=→"fancy circles":cluster{dbl[], dbl[]}[])  [unwired: 10 in]
